vi "Form Data Analysis.vi"(11 "表单数据":string) -> (2 "value":string[](array[string]), 3 "key":string[](array[string]))   [LabVIEW 2019, in "HTTP Server.lvlib"]
uses:
  HTTP Server.lvlib
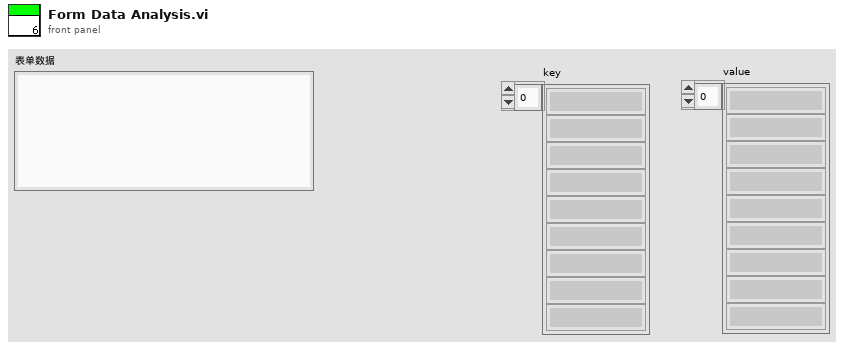
[diagram p1: front panel]
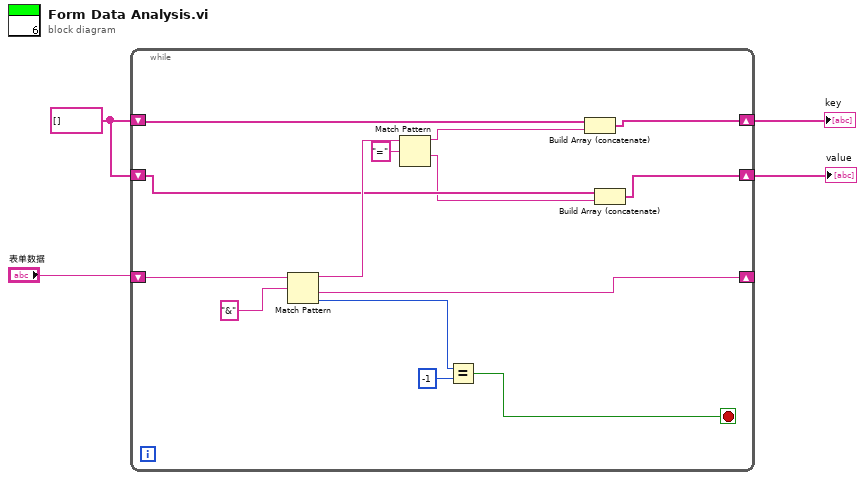
[diagram p0: block diagram]
diagram:
  w3 = string[] []
  n1 = while {
    shift-right: [w16] -> _
    shift-left: "表单数据" -> [w18]
    shift-right: [w6] -> w2
    shift-left: w3 -> [w10]
    shift-right: [w5] -> w1
    shift-left: w3 -> [w8]
    stop <- w13 stop-if-true
    n2 = Match Pattern(string=w18, regular expression="&" ("正则表达式")) -> (before substring=w12:string, after substring=w16:string, offset past match=w15:i32)  [unwired: 1 in, 1 out]
    n3 = Match Pattern(string=w12, regular expression="=" ("正则表达式")) -> (before substring=w9:string, after substring=w7:string)  [unwired: 1 in, 2 out]
    n4 = Equal?(x=w15, y=-1) -> (x = y?=w13:bool)
    n5 = Build Array (concatenate)(w10, w9) -> (w6:string[])
    n6 = Build Array (concatenate)(w8, w7) -> (w5:string[])
  }
  "key" <- w2
  "value" <- w1
